vi "lvcsm File Path.vi"() -> (1 "Appended Path":path)   [LabVIEW 2017, in "lvcsm File Support.lvlib"]
uses:
  lvcsm File Support.lvlib
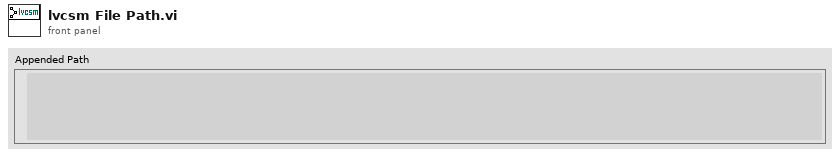
[diagram p1: front panel]
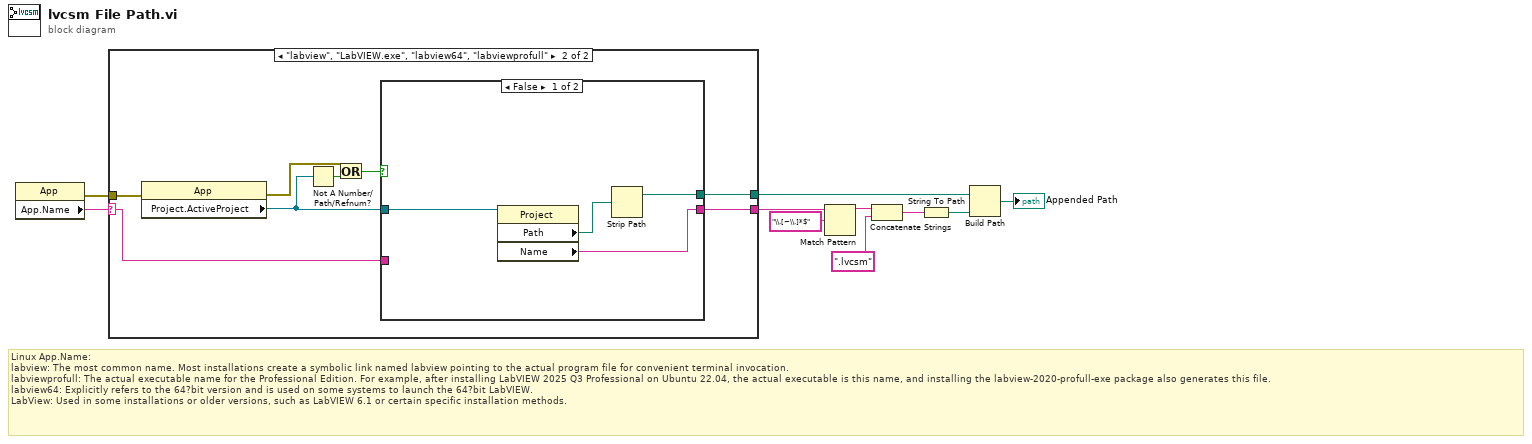
[diagram p0: block diagram]
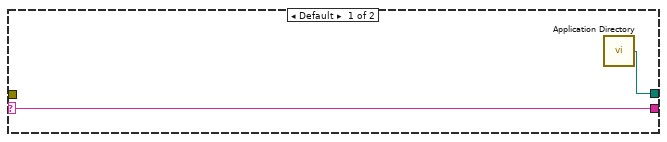
[diagram p2: hidden frame]
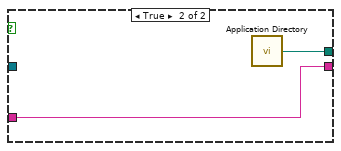
[diagram p3: hidden frame]
diagram:
  # "Linux App.Name:\nlabview: The most common name. Most installations create a symbolic link named labview pointing to the actual program file for convenient terminal invocation.\nlabviewprofull: The actual executable name for the Professional Edition. For example, after installing LabVIEW 2025 Q3 Professional on Ubuntu 22.04, the actual executable is this name, and installing the labview-2020-profull-exe package also generates this file.\nlabview64: Explicitly refers to the 64?bit version and is used on some systems to launch the 64?bit LabVIEW.\nLabView: Used in some installations or older versions, such as LabVIEW 6.1 or certain specific installation methods."
  n1 = property class="App"() -> (error out=w9:errorcluster, "App.Name"=w10:string)  [unwired: 2 in, 1 out]
  n2 = case shown="\"labview\", \"LabVIEW.exe\", \"labview64\", \"labviewprofull\"" w10 {
    selector: w10 -> [w12 w14]
    tunnel: w9 -> [_ w18]
    tunnel: [w12 w15] -> w7
    tunnel: [w11 w13] -> w2
    frame Default {
      n3 = call <vilib>:"Application Directory.vi"() -> ("Application Directory"=w11:path)
    }
    frame "labview", "LabVIEW.exe", "labview64", "labviewprofull" {
      n4 = property class="App"(error in=w18) -> (error out=w20:errorcluster, "Project.ActiveProject"=w17:refnum<vi>)  [unwired: 1 in, 1 out]
      n5 = Not A Number/Path/Refnum?(number/path/refnum=w17) -> (NaN/Path/Refnum?=w19:bool)
      n6 = Or(x=w20, y=w19) -> (x .or. y?=w16:bool)
      n7 = case shown="False" w16 {
        tunnel: w17 -> [w24 _]
        tunnel: [w23 w26] -> w15
        tunnel: w14 -> [_ w26]
        tunnel: [w21 w25] -> w13
        frame False {
          n8 = property class="Project"(reference=w24) -> ("Path"=w22:path, "Name"=w23:string)  [unwired: 1 in, 2 out]
          n9 = Strip Path(path=w22) -> (stripped path=w21:path)  [unwired: 1 out]
        }
        frame True {
          n10 = call <vilib>:"Application Directory.vi"() -> ("Application Directory"=w25:path)
        }
      }
    }
  }
  n11 = Match Pattern(string=w7, regular expression="\\.[~\\.]*$") -> (before substring=w5:string)  [unwired: 1 in, 3 out]
  n12 = Concatenate Strings(w5, ".lvcsm" ("new ending (none)")) -> (w4:string)
  n13 = String To Path(string=w4) -> (path=w1:path)
  n14 = Build Path(base path=w2, name or relative path=w1) -> (appended path=→"Appended Path":path)
